vi "CalculateSNR.vi"(2 "Original Signal":dbl[](array[numeric]), 3 "Sampled Signal":dbl[](array[numeric])) -> (1 "SNR":dbl)   [LabVIEW 2014]
uses:
  <vilib>/Analysis/baseanly.llb/Real Dot Product.vi
  <vilib>/Analysis/NI_AALBase.lvlib
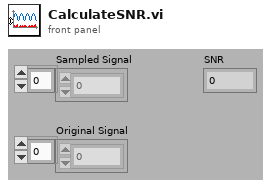
[diagram p1: front panel]
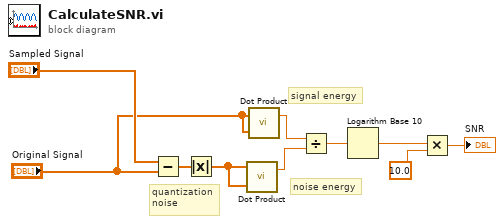
[diagram p0: block diagram]
diagram:
  # "signal energy"
  # "noise energy"
  # "quantization\nnoise"
  n1 = Subtract(x="Sampled Signal", y="Original Signal") -> (x-y=w4:dbl[])
  n2 = Absolute Value(x=w4) -> (abs(x)=w1:dbl[])
  n3 = call-poly <vilib>:"Dot Product.vi"("Y Vector"=w1, "X Vector"=w1) -> ("X * Y"=w10:dbl)  [unwired: 1 out]
  n4 = call-poly <vilib>:"Dot Product.vi"("Y Vector"="Original Signal", "X Vector"="Original Signal") -> ("X * Y"=w9:dbl)  [unwired: 1 out]
  n5 = Divide(x=w9, y=w10) -> (x/y=w8:dbl)
  n6 = Logarithm Base 10(1:w8) -> (0:w7:dbl)
  n7 = Multiply(x=w7, y=10.0) -> (x*y=→"SNR":dbl)
